vi "Get Error Log File Name.vi"(8 "error in (no error)":errorcluster, 10 "Extension":string, 11 "Error Log Path in":path) -> (0 "error out":errorcluster, 3 "Error Log Path out":path)   [LabVIEW 2020, in "Error Log Classes.lvlib" / "Error Log.lvclass"]
uses:
  Error Log.lvclass
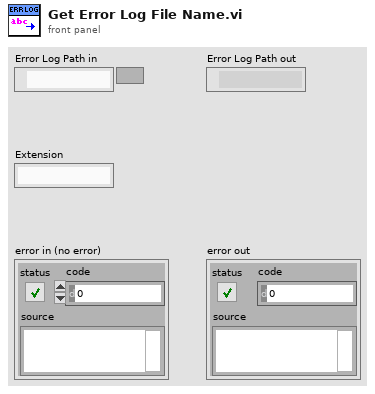
[diagram p1: front panel]
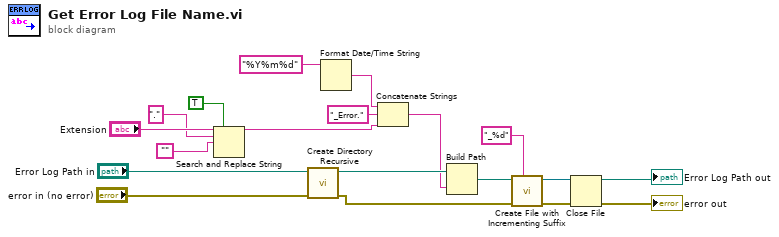
[diagram p0: block diagram]
diagram:
  n1 = Search and Replace String(replace all?=TRUE ("replace all? (F)"), input string="Extension", search string=".", replace string="") -> (result string=w12:string)  [unwired: 4 in, 3 out]
  n2 = call <vilib>:"Create Directory Recursive.vi"("error in (no error)"="error in (no error)", "directory"="Error Log Path in") -> ("error out"=w3:errorcluster, "directory copy"=w17:path)  [unwired: 3 in, 1 out]
  n3 = Format Date/Time String(time format string (%c)="%Y%m%d") -> (date/time string=w14:string)  [unwired: 2 in]
  n4 = Concatenate Strings(w14, "_Error." ("string"), w12) -> (w16:string)
  n5 = Build Path(base path=w17, name or relative path=w16) -> (appended path=w6:path)
  n6 = call <vilib>:"Create File with Incrementing Suffix.vi"("format string (\" (%d)\")"="_%d" ("format string (\" (%d)\")"), "error in (no error)"=w3, "file path"=w6) -> ("error out"=w2:errorcluster, "refnum out"=w4:refnum<file>)  [unwired: 6 in, 1 out]
  n7 = Close File(refnum=w4, error in=w2) -> (path=→"Error Log Path out":path, error out=→"error out":errorcluster)
